vi "Mute Single.vi"(8 "Error In":errorcluster, 9 "Mute":bool, 10 "Detector":u8, 11 "KIT-QVA in":refnum<class "KIT-QVA.lvclass">) -> (0 "Error Out":errorcluster, 3 "KIT-QVA out":refnum<class "KIT-QVA.lvclass">)   [LabVIEW 2015, in "KIT-QVA.lvlib" / "KIT-QVA.lvclass"]
doc: "Activate or deactivate time unlimited muting of selected detector."
uses:
  KIT-QVA.lvclass
  KIT-QVA.lvclass/KIT-QVA.ctl
  instr.lib/KIT-QV/KIT QV.lvlib
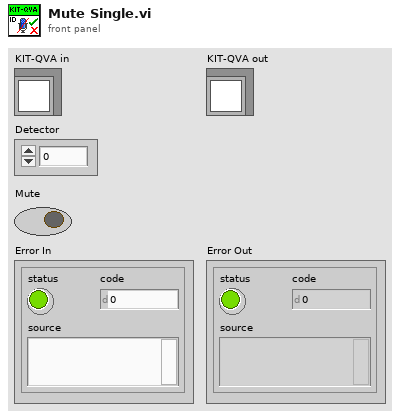
[diagram p1: front panel]
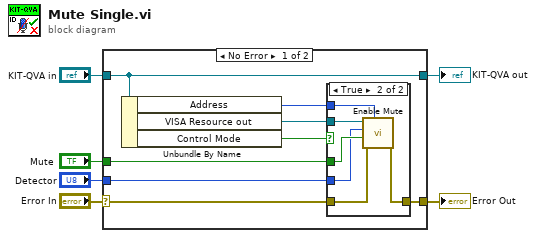
[diagram p0: block diagram]
diagram:
  n1 = case shown="No Error" "Error In" {
    selector: "Error In" -> [w11 w23]
    tunnel: [w10 w23] -> w5
    tunnel: [w14 w22] -> w3
    tunnel: "KIT-QVA in" -> [w14 w22]
    tunnel: "Mute" -> [w9 _]
    tunnel: "Detector" -> [w8 _]
    frame No Error {
      n2 = Unbundle By Name(w14) -> ("Address"=w12:u16, "VISA Resource out"=w13:refnum<visa-resource-name>, "Control Mode"=w7:bool)
      n3 = case shown="True" w7 {
        tunnel: w13 -> [_ w21]
        tunnel: w12 -> [_ w20]
        tunnel: w11 -> [w15 w19]
        tunnel: w9 -> [_ w17]
        tunnel: [w15 w18] -> w10
        tunnel: w8 -> [_ w16]
        frame False {
        }
        frame True {
          n4 = call "Enable Mute.vi"("Address"=w20, "Error In"=w19, "Mute (F)"=w17, "Detector"=w16, "VISA Resource in"=w21) -> ("Error Out"=w18:errorcluster)  [unwired: 5 in, 1 out]
        }
      }
    }
    frame Error {
    }
  }
  "Error Out" <- w5
  "KIT-QVA out" <- w3
